vi "Esercizio lezione 8-2 My Simple Client.vi"(1 "Server Address":string="localhost", 2 "Port":u16=6340 min=1025 step=1) -> (0 "read string":string)   [LabVIEW 2012]
doc: "© Copyright M. Ferrari 2010"
panel:
  # "CLIENT: legge una stringa inviata dal Server"
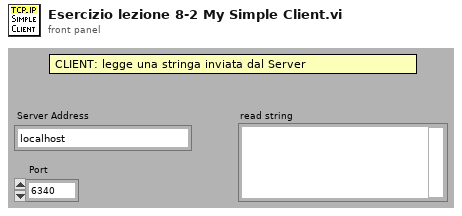
[diagram p1: front panel]
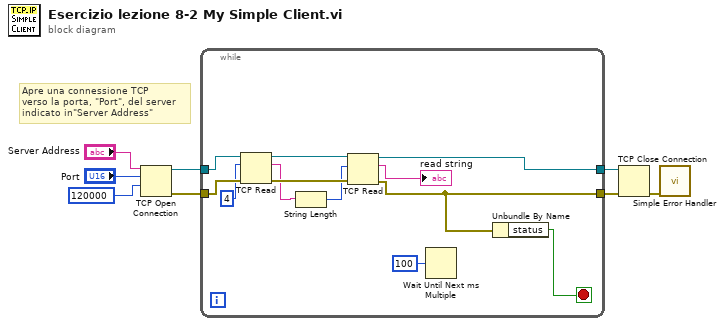
[diagram p0: block diagram]
diagram:
  # "Apre una connessione TCP\nverso la porta, \"Port\", del server\nindicato in\"Server Address\""
  n1 = TCP Open Connection(address="Server Address", remote port or service name="Port", timeout ms (60000)=120000) -> (connection ID=w5:refnum<k5>, error out=w6:errorcluster)  [unwired: 2 in]
  n2 = while {
    tunnel: w5 -> [w18]
    tunnel: w6 -> [w15]
    tunnel: [w10] -> w2
    tunnel: [w13] -> w1
    stop <- w19 stop-if-true
    n3 = TCP Read(connection ID=w18, bytes to read=4, error in (no error)=w15) -> (connection ID out=w16:refnum<k5>, data out=w9:string, error out=w14:errorcluster)  [unwired: 2 in]
    n4 = String Length(string=w9) -> (length=w12:i32)
    n5 = TCP Read(connection ID=w16, bytes to read=w12, error in (no error)=w14) -> (connection ID out=w10:refnum<k5>, data out=→"read string":string, error out=w13:errorcluster)  [unwired: 2 in]
    n6 = Wait Until Next ms Multiple(millisecond multiple=u32 100) -> ()  [unwired: 1 out]
    n7 = Unbundle By Name(w13) -> ("status"=w19:bool)
  }
  n8 = TCP Close Connection(connection ID=w2, error in (no error)=w1) -> (error out=w4:errorcluster)  [unwired: 1 in, 1 out]
  n9 = call <vilib>:"Simple Error Handler.vi"("error in (no error)"=w4) -> ()  [unwired: 4 in, 5 out]
